vi "配置信息读取.vi"(11 "被复制模型":cluster{"参数":u8, "测量模式":u8, "量程":u8}) -> (3 "输出簇":T2 {"曲线模型"."r^2" format="%.7g"})   [LabVIEW 2016, in "曲线模型.xctl"]
uses:
  <vilib>/Utility/config.llb/NI_LVConfig.lvlib
panel:
  # "标液浓度"
  # "F0"
  # "F1"
  # "吸光值显示"
  # "辅\n助\n计\n算\n区"
  # "样品一"
  # "样品二"
  # "样品三"
  # "样品四"
  # "样品五"
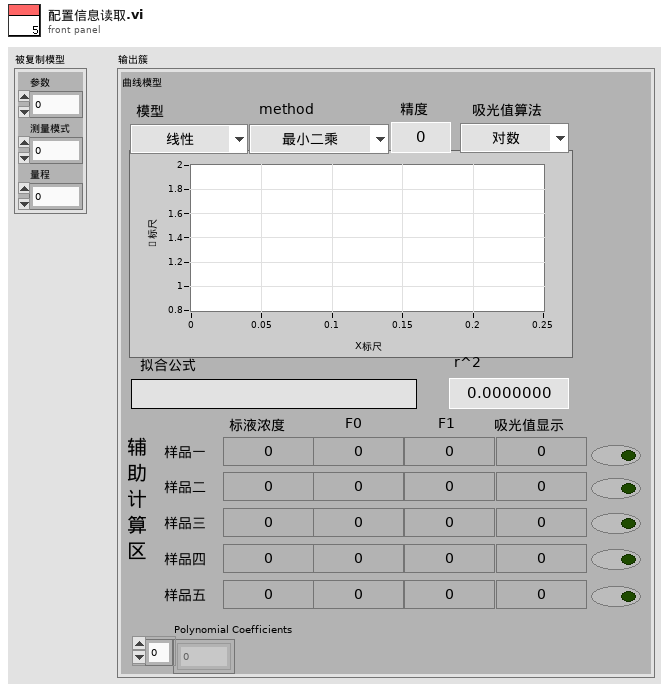
[diagram p1: front panel]
types:
  T1 = typedef "曲线模型.xctl/曲线模型外观.ctl" = cluster{"标液浓度1":dbl, "样品1 F0":dbl, "样品1 F1":dbl, "测量吸光度1":dbl, "样品1启用":bool, "标液浓度2":dbl, "样品2 F0":dbl, "样品2 F1":dbl, "测量吸光度2":dbl, "样品2启用":bool, "标液浓度3":dbl, "样品3 F0":dbl, "样品3 F1":dbl, "测量吸光度3":dbl, "样品3启用":bool, "标液浓度4":dbl, "样品4 F0":dbl, "样品4 F1":dbl, "测量吸光度4":dbl, "样品4启用":bool, "标液浓度5":dbl, "样品5 F0":dbl, "样品5 F1":dbl, "测量吸光度5":dbl, "样品5启用":bool, "模型":enum32{"线性", "多项式"}, "method":enum16{"最小二乘", "最小绝对残差", "Bisquare"}, "精度":dbl, "XY图":cluster{"X Values":dbl[], "Y Values":dbl[]}[], "拟合公式":string, "r^2":dbl, "吸光值算法":enum16{"对数", "减法"}}
  T2 = cluster{"曲线模型":T1, "Polynomial Coefficients":dbl[]}
  T3 = typedef "NI_LVConfig.lvlib/Config Data RefNum.ctl" = refnum<k1>
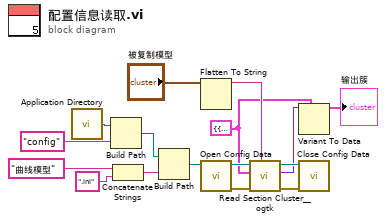
[diagram p0: block diagram]
diagram:
  w1 = T2 {"曲线模型"={"标液浓度1"=0.0, "样品1 F0"=0.0, "样品1 F1"=0.0, "测量吸光度1"=0.0, "样品1启用"=FALSE, "标液浓度2"=0.0, "样品2 F0"=0.0, "样品2 F1"=0.0, "测量吸光度2"=0.0, "样品2启用"=FALSE, "标液浓度3"=0.0, "样品3 F0"=0.0, "样品3 F1"=0.0, "测量吸光度3"=0.0, "样品3启用"=FALSE, "标液浓度4"=0.0, "样品4 F0"=0.0, "样品4 F1"=0.0, "测量吸光度4"=0.0, "样品4启用"=FALSE, "标液浓度5"=0.0, "样品5 F0"=0.0, "样品5 F1"=0.0, "测量吸光度5"=0.0, "样品5启用"=FALSE, "模型"=enum."线性", "method"=enum."最小二乘", "精度"=4.0, "XY图"=[], "拟合公式"="", "r^2"=0.0, "吸光值算法"=enum."对数"}, "Polynomial Coefficients"=[]} ("输出簇")
  n1 = call <vilib>:"Application Directory.vi"() -> ("Application Directory"=w9:path)
  n2 = Build Path(base path=w9, name or relative path="config" ("名称或相对路径")) -> (appended path=w7:path)
  n3 = Concatenate Strings("曲线模型" ("字符串"), ".ini" ("字符串")) -> (w5:string)
  n4 = Build Path(base path=w7, name or relative path=w5) -> (appended path=w10:path)
  n5 = Flatten To String(anything="被复制模型") -> (data string=w3:string)  [unwired: 3 in, 2 out]
  n6 = call <vilib>:"Open Config Data.vi"("configuration file path"=w10) -> ("error out"=w13:errorcluster, "refnum"=w14:T3)  [unwired: 8 in, 1 out]
  n7 = call <userlib>:"Read Section Cluster__ogtk.vi"("section (optional)"=w3, "error in (no error)"=w13, "Section Formatted Cluster Type"=w1, "refnum"=w14) -> ("error out"=w11:errorcluster, "Section Formatted Cluster"=w4:variant, "dup refnum"=w12:T3)  [unwired: 3 in, 2 out]
  n8 = Variant To Data(type=w1, Variant=w4) -> (data=→"输出簇":T2)  [unwired: 1 in, 1 out]
  n9 = call <vilib>:"Close Config Data.vi"("error in (no error)"=w11, "refnum"=w12) -> ()  [unwired: 8 in, 2 out]
